vi "From JSON.vi"(8 "error in (no error)":errorcluster, 10 "JSON":string, 11 "Double Float in":refnum<class "Abs_U32 Integer.lvclass">) -> (0 "error out":errorcluster, 3 "Double Float out":refnum<class "Abs_U32 Integer.lvclass">)   [LabVIEW 2021, in "Abs_U32 Integer.lvclass"]
uses:
  Abs_U32 Integer.lvclass
  C:/Program Files (x86)/National Instruments/LabVIEW 2021/vi.lib/TSA/Abstract Data Classes/Abs_Types/Type/Abs_Type.lvclass
  5ce128e4-fa1c-4878-9809-5fc217d2855a.vi
  <vilib>/JDP Science/JSONtext/Find Item.vi
  <vilib>/JDP Science/JSONtext/Next JSON Value.vi
  <vilib>/JDP Science/JSONtext/String Subset.vi
  <vilib>/JDP Science/JSONtext/Parsing/Advance past next JSON Value (inlined COPY).vi
  <vilib>/JDP Science/JSONtext/Parsing/Advance past whitespace.vi
  <vilib>/JDP Science/JSONtext/Parsing/Advance past String.vi
  <vilib>/JDP Science/JSONtext/Parsing/Advance past Number.vi
  <vilib>/JDP Science/JSONtext/Parsing/Advance past Line Ending.vi
  <vilib>/Utility/LVClass/Get LV Class Name.vi
  <vilib>/JDP Science/JSONtext/Parsing/Parse Full Path or Item Name.vi
  <vilib>/JDP Science/JSONtext/Parsing/Advance past Array.vi
  <vilib>/JDP Science/JSONtext/Parsing/Advance past Object.vi
  <vilib>/JDP Science/JSONtext/support/Error Cluster From Code.vi
  <vilib>/JDP Science/JSONtext/Offset/Find Item Locations by Path.vi
  <vilib>/JDP Science/JSONtext/JSON text to Variant.vi
  <vilib>/JDP Science/JSONtext/LVClass Serializer/JSONtext LVClass Serializer.lvclass
  Integer/Abs_Integer.lvclass
  Type/Abs_Type.lvclass
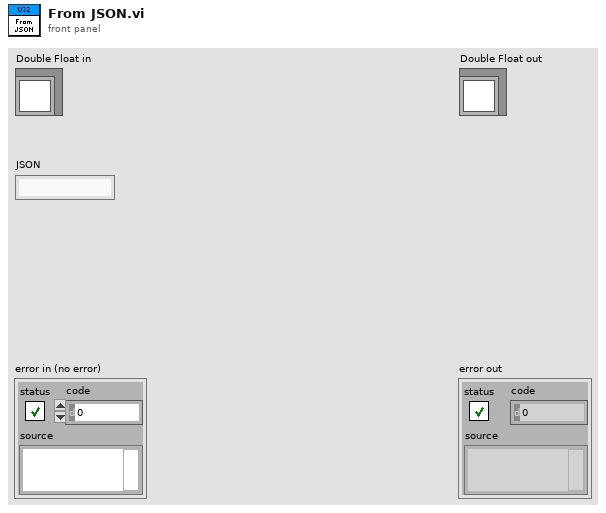
[diagram p1: front panel]
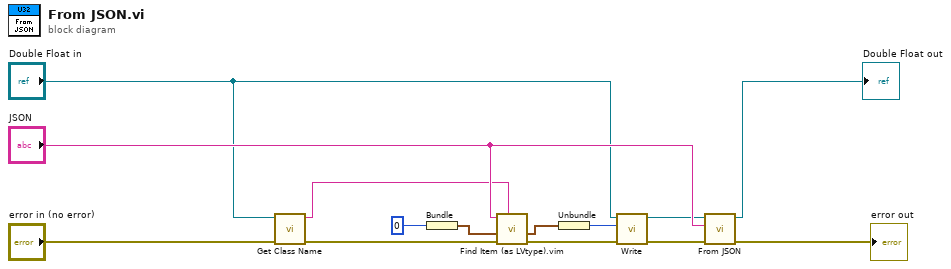
[diagram p0: block diagram]
diagram:
  n1 = call "Get Class Name.vi"("error in (no error)"="error in (no error)", "Abs_Type in"="Double Float in") -> ("error out"=w6:errorcluster, "class name"=w7:string)  [unwired: 8 in]
  n2 = Bundle("Value"=u32 0) -> (w8:cluster{"Value":u32})  [unwired: 1 in]
  n3 = call "Find Item (as LVtype).vim"("$Path or Item Name"=w7, "error in (no error)"=w6, "Data Type and Default Value"=w8, "JSON"="JSON") -> ("error out"=w5:errorcluster, "Data"=w9:cluster{"Value":u32})  [unwired: 4 in, 2 out]
  n4 = Unbundle(w9) -> ("Value"=w2:u32)
  n5 = call-dynamic "Write.vi"("error in (no error)"=w5, "Value"=w2, "Double Float.lvclass_340760 in"="Double Float in") -> ("error out"=w4:errorcluster, "Double Float.lvclass_340760 out"=w3:refnum<class "Abs_U32 Integer.lvclass">)  [unwired: 7 in]
  n6 = call-parent "From JSON.vi"("error in (no error)"=w4, "JSON"="JSON", "Type in"=w3) -> ("error out"=→"error out":errorcluster, "Type out"=→"Double Float out":refnum<class "Abs_U32 Integer.lvclass">)  [unwired: 7 in]
